vi "tell current position.vi"(6 "error in":errorcluster, 8 "Axis in":i32=1, 9 "VISA Handle in":refnum<visa-resource-name>) -> (0 "error out":errorcluster, 1 "Current position (units)":dbl format="%.2f", 2 "Axis out":i32=1, 3 "VISA Handle out":refnum<visa-resource-name>, 4 "TimeoutFlag":bool)   [LabVIEW 2018]
doc: "This VI returns the current position. This is the encoder feedback position. This position will always change."
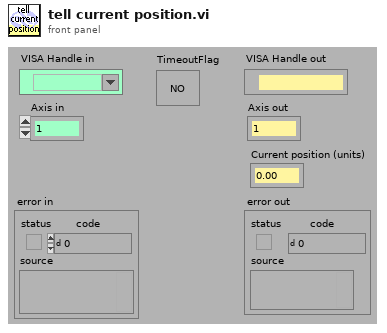
[diagram p1: front panel]
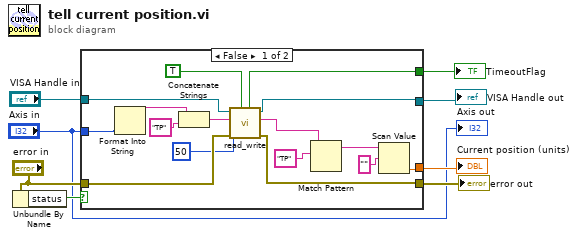
[diagram p0: block diagram]
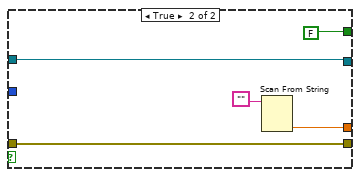
[diagram p2: hidden frame]
diagram:
  n1 = Unbundle By Name("error in") -> ("status"=w6:bool)
  n2 = case shown="False" w6 {
    tunnel: [w20 w29] -> w8
    tunnel: [w13 w26] -> w2
    tunnel: [w19 w28] -> w7
    tunnel: "VISA Handle in" -> [w23 w29]
    tunnel: "error in" -> [w21 w28]
    tunnel: [w18 FALSE ("TimeoutFlag")] -> w3
    tunnel: "Axis in" -> [w10 _]
    frame False {
      n3 = Format Into String(w10) -> (resulting string=w16:string)  [unwired: 3 in, 1 out]
      n4 = Concatenate Strings(w16, "TP" ("string")) -> (w22:string)
      n5 = call "read_write.vi"("Query?"=TRUE, "error in"=w21, "Bytes to read"=50, "Command"=w22, "VISA handle in"=w23) -> ("error out"=w19:errorcluster, "Response"=w15:string, "VISA handle out"=w20:refnum<visa-resource-name>, "TimeoutFlag"=w18:bool)  [unwired: 1 in]
      n6 = Match Pattern(string=w15, regular expression="TP" ("expression")) -> (after substring=w12:string)  [unwired: 1 in, 3 out]
      n7 = Scan Value(string=w12, format string="" ("chaîne de format")) -> (value=w13:dbl)  [unwired: 1 in, 1 out]
    }
    frame True {
      n8 = Scan From String(input string="") -> (output 1=w26:dbl)  [unwired: 4 in, 3 out]
    }
  }
  "VISA Handle out" <- w8
  "error out" <- w7
  "TimeoutFlag" <- w3
  "Current position (units)" <- w2
  "Axis out" <- "Axis in"
